vi "CutArray.vi"(0 "array":i8[](array[numeric]), 2 "From index":i32, 3 "Length":i32) -> (5 "Sub array":i8[](array[numeric]))   [LabVIEW 2012]
doc: "Discards bits before \"From index\" and returns the following \"Length\" bits.\nI.e \"Sub array\" will consist of bits from \"from index\" to \"from index + length\"."
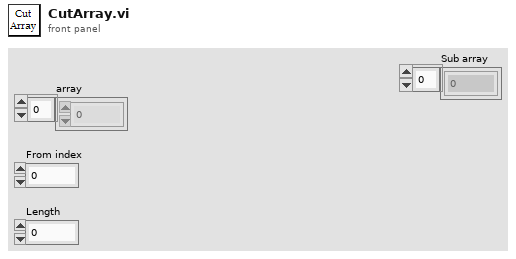
[diagram p1: front panel]
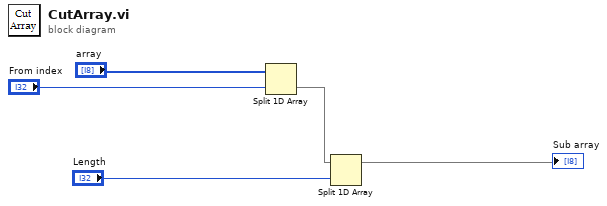
[diagram p0: block diagram]
diagram:
  n1 = Split 1D Array(array="array", index="From index") -> (second subarray=w4:i8[])  [unwired: 1 out]
  n2 = Split 1D Array(array=w4, index="Length") -> (first subarray=→"Sub array":i8[])  [unwired: 1 out]
